vi "Send TCP Message.vi"(3 "Error In":errorcluster, 4 "TCP Network Connection Refnum":refnum<k5>, 5 "Supervisor in":refnum<class "Supervisor.lvclass">) -> (0 "Error Out":errorcluster, 1 "TCP Network Connection Refnum Out":refnum<k5>, 2 "Supervisor out":refnum<class "Supervisor.lvclass">)   [LabVIEW 2014, in "Supervisor.lvclass"]
uses:
  Supervisor.lvclass
  Supervisor.lvclass/Supervisor.ctl
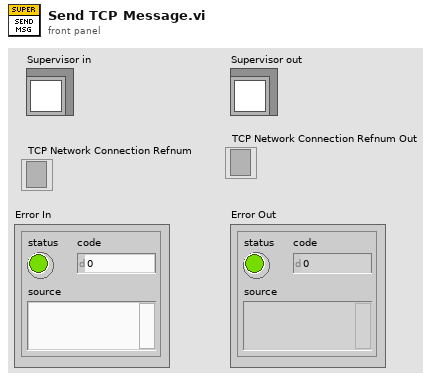
[diagram p1: front panel]
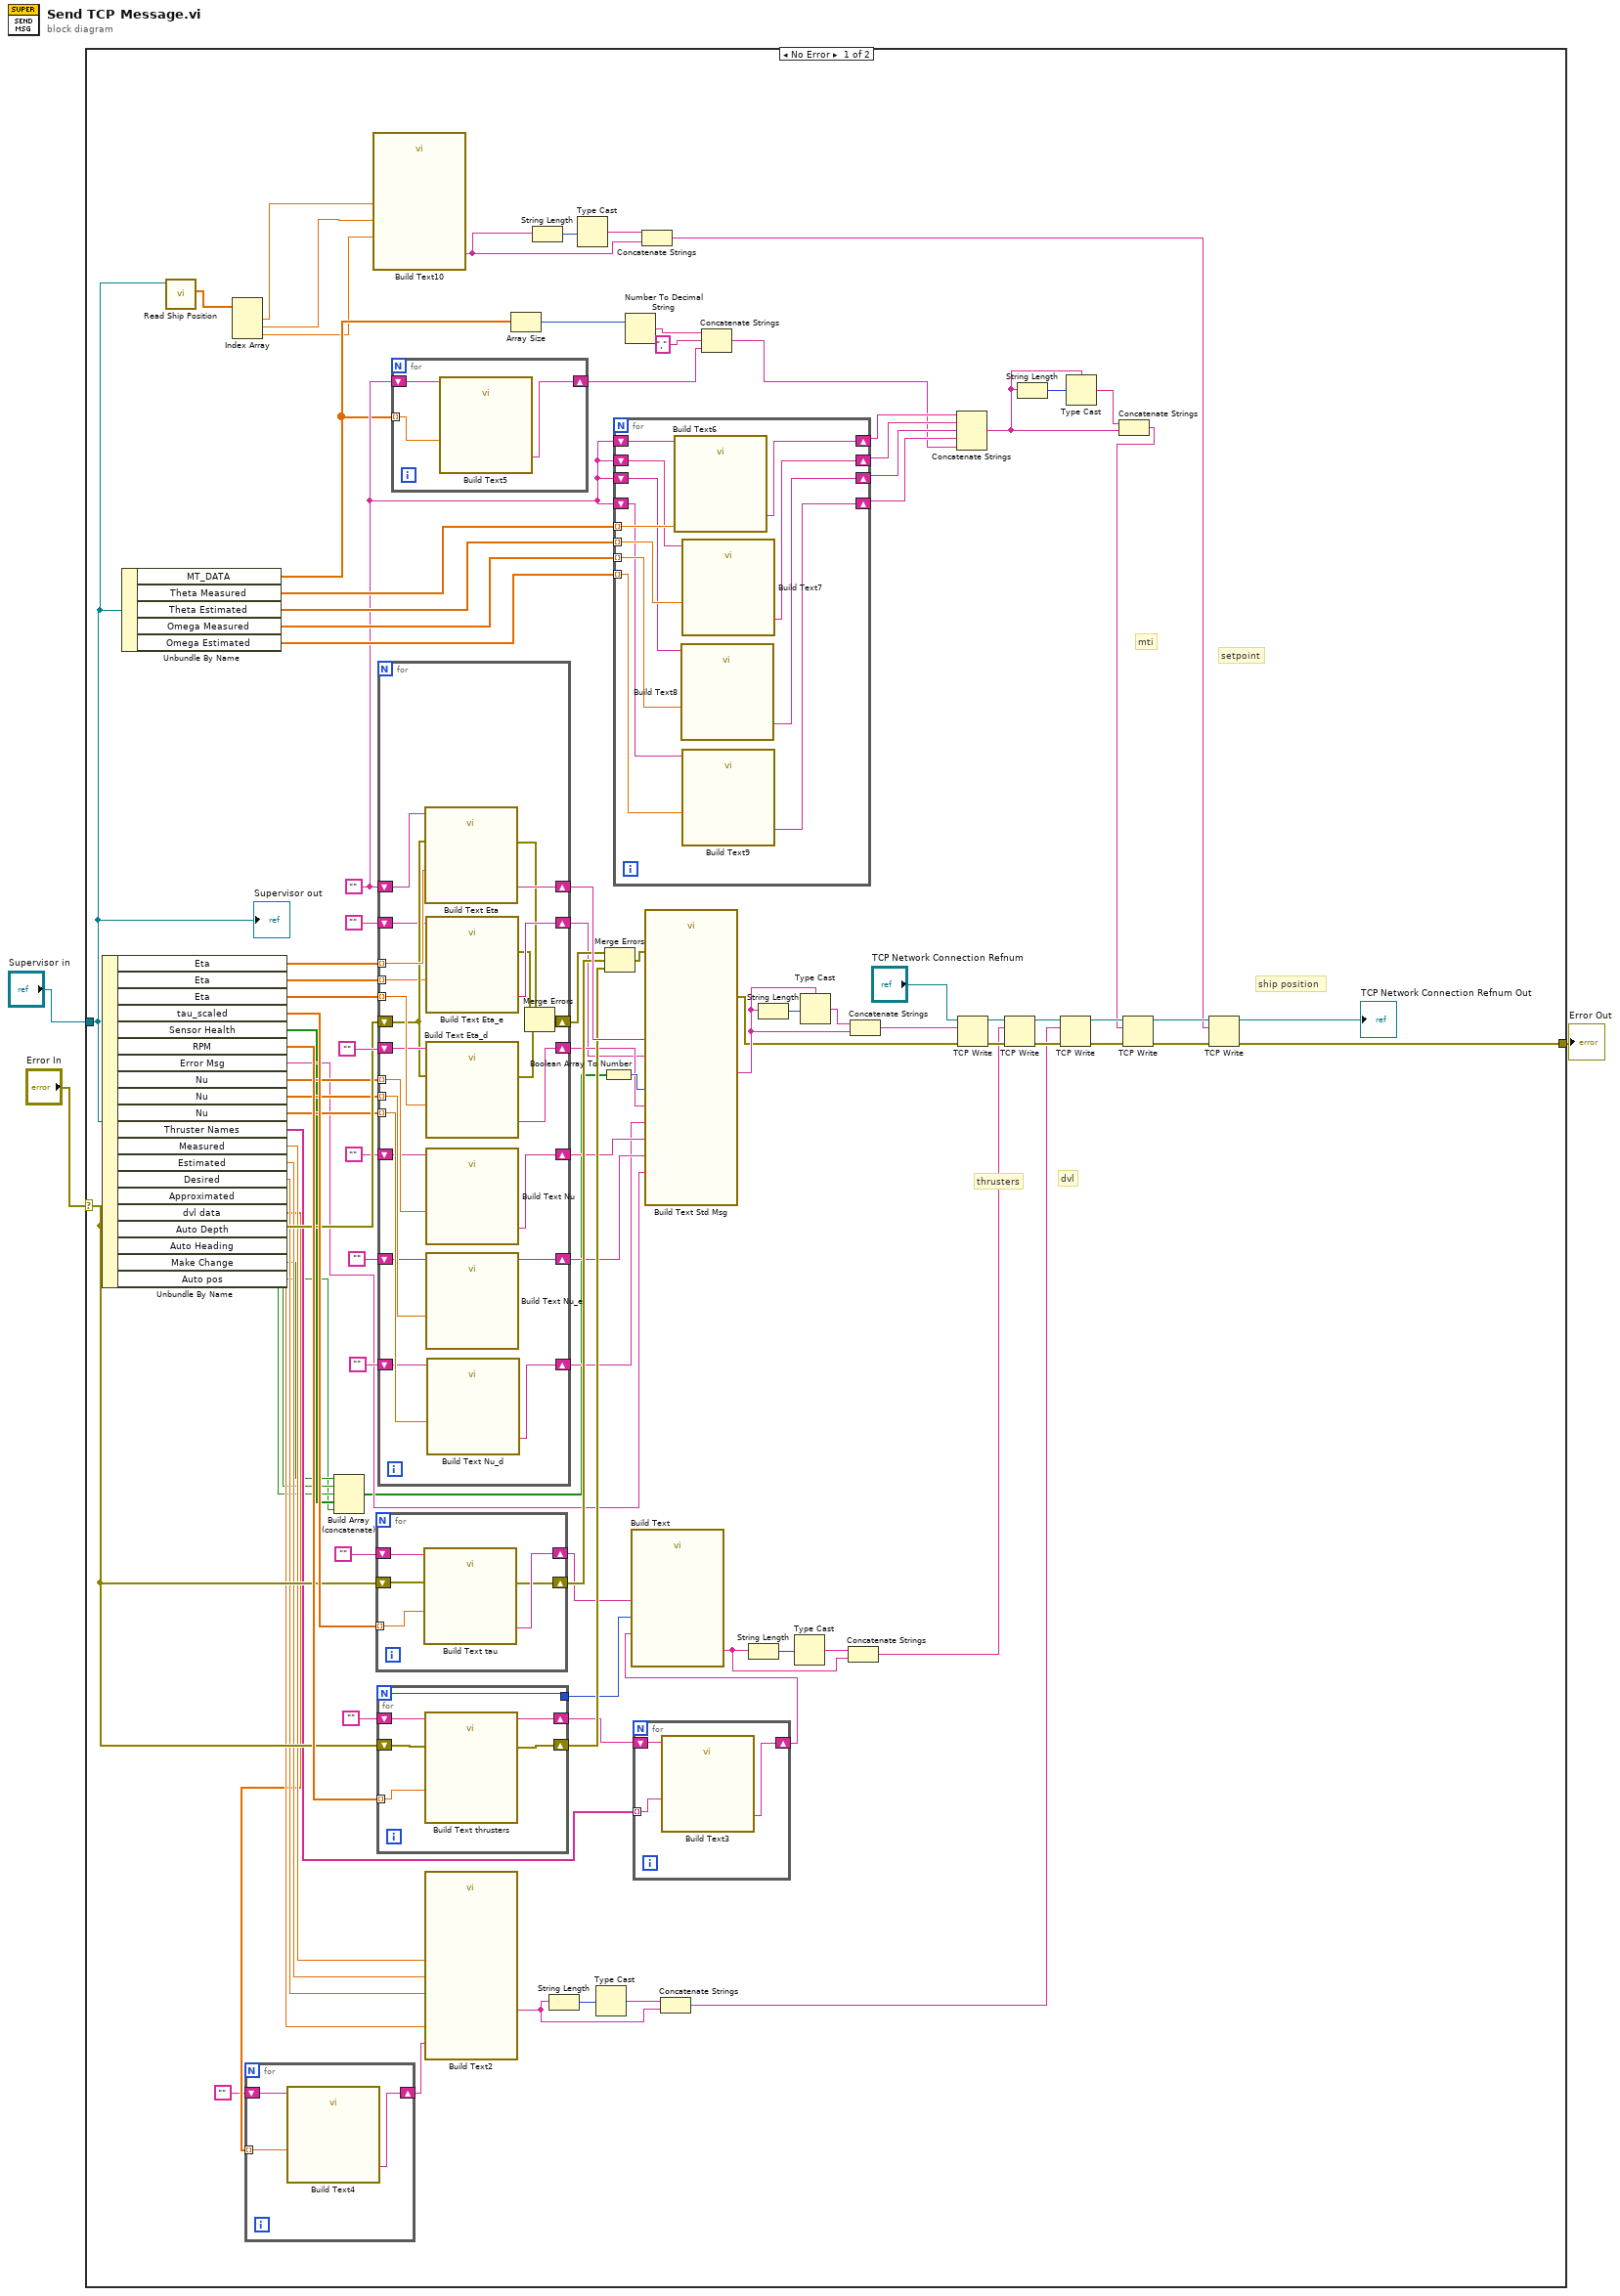
[diagram p0: block diagram]
diagram:
  n1 = case shown="No Error" "Error In" {
    selector: "Error In" -> [w90 w157]
    tunnel: "Supervisor in" -> [w10 _]
    tunnel: [w4 w157] -> w1
    frame No Error {
      w30 = ""
      # "setpoint"
      # "mti"
      # "dvl"
      # "thrusters"
      # "ship position"
      n2 = Unbundle By Name(w10) -> ("Eta"=w82:dbl[], "Eta"=w81:dbl[], "Eta"=w101:dbl[], "tau_scaled"=w94:dbl[], "Sensor Health"=w50:bool[], "RPM"=w92:dbl[], "Error Msg"=w72:string, "Nu"=w78:dbl[], "Nu"=w77:dbl[], "Nu"=w76:dbl[], "Thruster Names"=w57:string[], "Measured"=w63:dbl, "Estimated"=w62:dbl, "Desired"=w61:dbl, "Approximated"=w54:dbl, "dvl data"=w53:dbl[], "Auto Depth"=w48:bool, "Auto Heading"=w47:bool, "Make Change"=w46:bool, "Auto pos"=w11:bool)
      n3 = Unbundle By Name(w10) -> ("MT_DATA"=w23:dbl[], "Theta Measured"=w38:dbl[], "Theta Estimated"=w37:dbl[], "Omega Measured"=w36:dbl[], "Omega Estimated"=w35:dbl[])
      n4 = call-dynamic "Read Ship Position.vi"("Supervisor in"=w10) -> ("Ship Position"=w9:dbl[])  [unwired: 8 in, 2 out]
      n5 = Index Array(array=w9) -> (element #1=w8:dbl, element #2=w7:dbl, element #3=w6:dbl)  [unwired: 3 in]
      n6 = for {
        tunnel: w53 -> [w119] mode=indexing
        shift-right: [w118] -> w51
        shift-left: "" -> [w117]
        n7 = call "Build Text4"("Beginning Text"=w117, "Value"=w119) -> ("Result"=w118:string)  [unwired: 12 in, 1 out]
      }
      n8 = Build Array (concatenate)(w46, w48, w47, w50, w11) -> (w49:bool[])
      n9 = call "Build Text10"("North"=w8, "East"=w7, "Heading"=w6) -> ("Result"=w15:string)  [unwired: 11 in, 1 out]
      n10 = for {
        tunnel: w94 -> [w132] mode=indexing
        shift-right: [w131] -> w68
        shift-left: "" -> [w133]
        shift-right: [w129] -> w86
        shift-left: w90 -> [w130]
        n11 = call "Build Text tau"("Beginning Text"=w133, "Value"=w132, "error in (no error)"=w130) -> ("Result"=w131:string, "error out"=w129:errorcluster)  [unwired: 11 in]
      }
      n12 = for {
        N -> [w124]
        tunnel: w92 -> [w123] mode=indexing
        shift-right: [w127] -> w56
        shift-left: "" -> [w128]
        shift-right: [w125] -> w85
        shift-left: w90 -> [w126]
        tunnel: [w124] -> w67
        n13 = call "Build Text thrusters"("Beginning Text"=w128, "Value"=w123, "error in (no error)"=w126) -> ("Result"=w127:string, "error out"=w125:errorcluster)  [unwired: 11 in]
      }
      n14 = for {
        tunnel: w82 -> [w156] mode=indexing
        tunnel: w101 -> [w155] mode=indexing
        shift-right: [w154] -> w83
        shift-left: "" -> [w153]
        shift-right: [w152] -> w99
        shift-left: w30 -> [w151]
        shift-right: [w148] -> w87
        shift-left: w90 -> [w150]
        tunnel: w81 -> [w147] mode=indexing
        shift-right: [w146] -> w79
        shift-left: "" -> [w145]
        tunnel: w78 -> [w142] mode=indexing
        tunnel: w77 -> [w141] mode=indexing
        tunnel: w76 -> [w140] mode=indexing
        shift-right: [w139] -> w70
        shift-left: "" -> [w138]
        shift-right: [w137] -> w71
        shift-left: "" -> [w136]
        shift-right: [w135] -> w69
        shift-left: "" -> [w134]
        n15 = call "Build Text Eta"("Beginning Text"=w151, "Value"=w156, "error in (no error)"=w150) -> ("Result"=w152:string, "error out"=w144:errorcluster)  [unwired: 11 in]
        n16 = call "Build Text Eta_e"("Beginning Text"=w145, "Value"=w147) -> ("Result"=w146:string, "error out"=w143:errorcluster)  [unwired: 12 in]
        n17 = call "Build Text Eta_d"("Beginning Text"=w153, "Value"=w155, "error in (no error)"=w150) -> ("Result"=w154:string, "error out"=w149:errorcluster)  [unwired: 11 in]
        n18 = call "Build Text Nu"("Beginning Text"=w136, "value"=w142) -> ("Result"=w137:string)  [unwired: 12 in, 1 out]
        n19 = call "Build Text Nu_e"("Beginning Text"=w138, "value"=w141) -> ("Result"=w139:string)  [unwired: 12 in, 1 out]
        n20 = call "Build Text Nu_d"("Beginning Text"=w134, "value"=w140) -> ("Result"=w135:string)  [unwired: 12 in, 1 out]
        n21 = Merge Errors(w144, w143, w149) -> (w148:errorcluster)
      }
      n22 = for {
        tunnel: w23 -> [w116] mode=indexing
        shift-right: [w115] -> w19
        shift-left: w30 -> [w114]
        n23 = call "Build Text5"("Beginning Text"=w114, "Value"=w116) -> ("Result"=w115:string)  [unwired: 12 in, 1 out]
      }
      n24 = call "Build Text2"("Approximated"=w54, "Measured"=w63, "Estimated"=w62, "Desired"=w61, "DVL"=w51) -> ("Result"=w58:string)  [unwired: 9 in, 1 out]
      n25 = Array Size(array=w23) -> (size(s)=w22:i32)
      n26 = String Length(string=w15) -> (length=w17:i32)
      n27 = String Length(string=w58) -> (length=w60:i32)
      n28 = Type Cast(x=w17) -> (*(type *) &x=w16:string)  [unwired: 1 in]
      n29 = Type Cast(x=w60) -> (*(type *) &x=w59:string)  [unwired: 1 in]
      n30 = Boolean Array To Number(Boolean array=w49) -> (number=w84:u32)
      n31 = Merge Errors(w87, w86, w85) -> (w89:errorcluster)
      n32 = for {
        tunnel: w38 -> [w113] mode=indexing
        tunnel: w37 -> [w110] mode=indexing
        tunnel: w36 -> [w107] mode=indexing
        tunnel: w35 -> [w104] mode=indexing
        shift-right: [w112] -> w34
        shift-left: w30 -> [w111]
        shift-right: [w109] -> w33
        shift-left: w30 -> [w108]
        shift-right: [w106] -> w32
        shift-left: w30 -> [w105]
        shift-right: [w103] -> w31
        shift-left: w30 -> [w102]
        n33 = call "Build Text6"("Beginning Text"=w111, "Value"=w113) -> ("Result"=w112:string)  [unwired: 12 in, 1 out]
        n34 = call "Build Text8"("Beginning Text"=w105, "Value"=w107) -> ("Result"=w106:string)  [unwired: 12 in, 1 out]
        n35 = call "Build Text7"("Beginning Text"=w108, "Value"=w110) -> ("Result"=w109:string)  [unwired: 12 in, 1 out]
        n36 = call "Build Text9"("Beginning Text"=w102, "Value"=w104) -> ("Result"=w103:string)  [unwired: 12 in, 1 out]
      }
      n37 = Number To Decimal String(number=w22) -> (decimal integer string=w21:string)  [unwired: 1 in]
      n38 = for {
        tunnel: w57 -> [w122] mode=indexing
        shift-right: [w120] -> w55
        shift-left: w56 -> [w121]
        n39 = call "Build Text3"("Beginning Text"=w121, "Name"=w122) -> ("Result"=w120:string)  [unwired: 12 in, 1 out]
      }
      n40 = call "Build Text"("tau"=w68, "num_thrusters"=w67, "thrusters"=w55) -> ("Result"=w64:string)  [unwired: 11 in, 1 out]
      n41 = Concatenate Strings(w16, w15) -> (w12:string)
      n42 = call "Build Text Std Msg"("Sensor_Status"=w84, "Nu_est"=w70, "Error_Msg"=w72, "Eta"=w99, "Eta_est"=w79, "Eta_d"=w83, "error in (no error)"=w89, "Nu"=w71, "Nu_d"=w69) -> ("Result"=w96:string, "error out"=w88:errorcluster)  [unwired: 5 in]
      n43 = Concatenate Strings(w59, w58) -> (w39:string)
      n44 = Concatenate Strings(w21, ",", w19) -> (w18:string)
      n45 = String Length(string=w64) -> (length=w66:i32)
      n46 = String Length(string=w96) -> (length=w98:i32)
      n47 = Type Cast(x=w66) -> (*(type *) &x=w65:string)  [unwired: 1 in]
      n48 = Type Cast(type=w96, x=w98) -> (*(type *) &x=w97:string)
      n49 = Concatenate Strings(w65, w64) -> (w40:string)
      n50 = Concatenate Strings(w97, w96) -> (w95:string)
      n51 = Concatenate Strings(w34, w33, w32, w31, w18) -> (w27:string)
      n52 = TCP Write(connection ID="TCP Network Connection Refnum", data in=w95, error in (no error)=w88) -> (connection ID out=w45:refnum<k5>, error out=w42:errorcluster)  [unwired: 1 in, 1 out]
      n53 = TCP Write(connection ID=w45, data in=w40, error in (no error)=w42) -> (connection ID out=w44:refnum<k5>, error out=w41:errorcluster)  [unwired: 1 in, 1 out]
      n54 = String Length(string=w27) -> (length=w29:i32)
      n55 = TCP Write(connection ID=w44, data in=w39, error in (no error)=w41) -> (connection ID out=w26:refnum<k5>, error out=w25:errorcluster)  [unwired: 1 in, 1 out]
      n56 = Type Cast(type=w27, x=w29) -> (*(type *) &x=w28:string)
      n57 = Concatenate Strings(w28, w27) -> (w24:string)
      n58 = TCP Write(connection ID=w26, data in=w24, error in (no error)=w25) -> (connection ID out=w14:refnum<k5>, error out=w13:errorcluster)  [unwired: 1 in, 1 out]
      n59 = TCP Write(connection ID=w14, data in=w12, error in (no error)=w13) -> (connection ID out=→"TCP Network Connection Refnum Out":refnum<k5>, error out=w4:errorcluster)  [unwired: 1 in, 1 out]
      "Supervisor out" <- w10
    }
    frame Error {
    }
  }
  "Error Out" <- w1
